vi "GEA3 Write ERD (Rev 2 API).vi"(0 "GEA2 Reference In":refnum<k24>, 1 "# of Tries":u8=5 min=1 step=1, 2 "Read Timeout (ms)":u32=500, 5 "GEA Inputs":T3 {"Destination" format="%.0x"; "Source" format="%.0x"}, 7 "ERD Write Data In":T1 {"ERD Number" format="%.0x"}, 11 "Error In":errorcluster, 13 "Verify ERD Response?":bool=TRUE) -> (4 "GEA2 Reference Out":refnum<k24>, 6 "Raw Data Out":string, 15 "Error Out":errorcluster)   [LabVIEW 2018, in "GEA2_Toolkit.lvlib"]
doc: "This VI writes an array of ERDs with a single command. The data type is used to convert the Data from the type specified to a hexidecimal string before sending it."
uses:
  C:/Users/iallatyp/Desktop/New folder/GEA3/library/GEA2_Toolkit.lvlib
  D:/Common/LabVIEW GEA2 Toolkit/source/GEA3 DLL Source/GeaCommunication.dll
  source/GEA3 DLL Source/GeaCommunication.dll
  type defs/Source_Destination.ctl
  type defs/ERD Write Data In.ctl
  type defs/Data Type.ctl
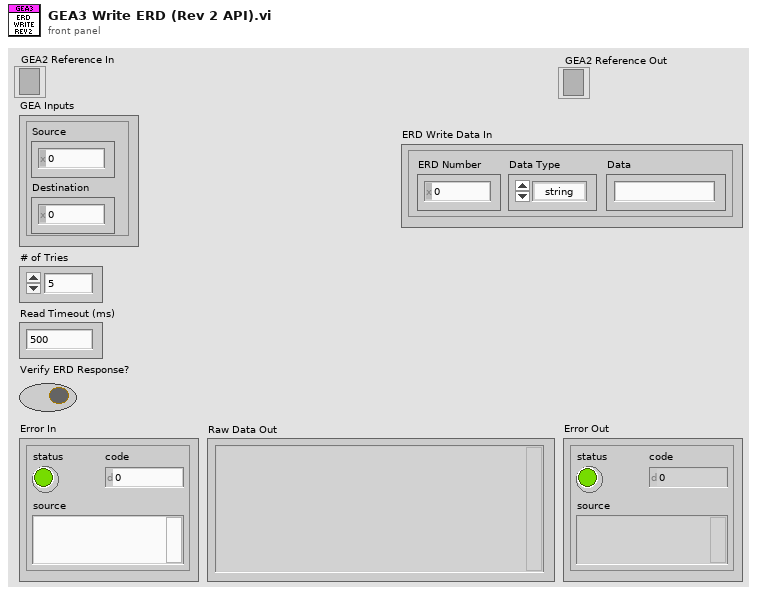
[diagram p1: front panel]
types:
  T1 = typedef "GEA2_Toolkit.lvlib/ERD Write Data In.ctl" = cluster{"ERD Number":u16, "Data Type":T2, "Data":string}
  T2 = typedef "GEA2_Toolkit.lvlib/Data Type.ctl" = enum16{"string", "boolean", "uint8_t", "uint16_t", "uint32_t", "uint64_t", "int8_t", "int16_t", "int32_t", "int64_t"}
  T3 = typedef "GEA2_Toolkit.lvlib/Source_Destination.ctl" = cluster{"Source":u8, "Destination":u8}
  T4 = typedef "GEA2_Toolkit.lvlib/Data In.ctl" = cluster{"Source":u8, "Destination":u8, "Command":u8, "Message":string}
  T5 = typedef "GEA2_Toolkit.lvlib/Data Out.ctl" = cluster{"Source":u8, "Destination":u8, "Command":u8, "Length":u8, "CRC":u16, "Message":string}
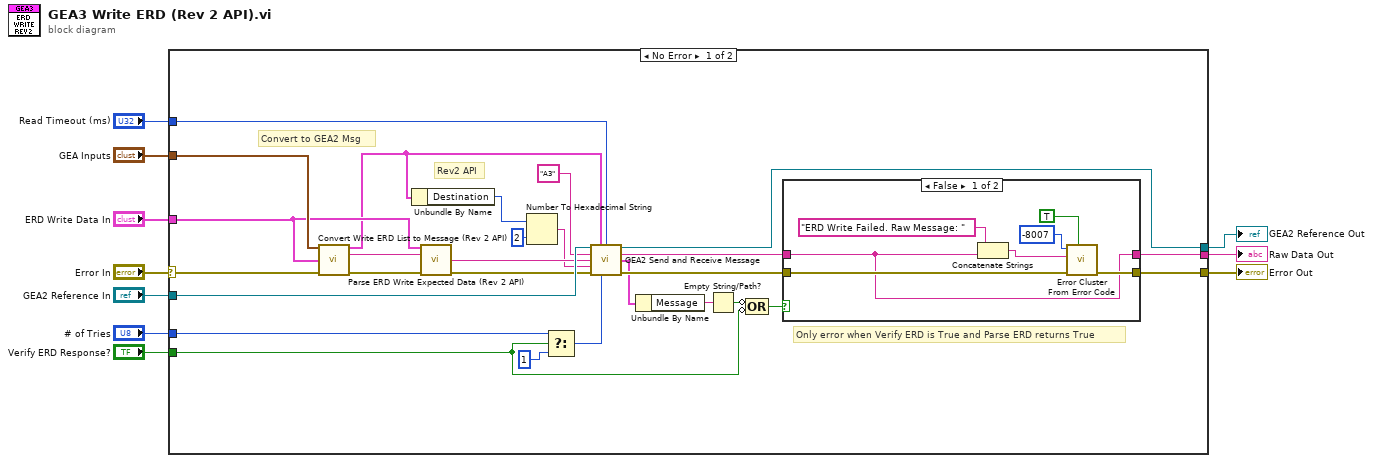
[diagram p0: block diagram]
diagram:
  n1 = case shown="No Error" "Error In" {
    selector: "Error In" -> [w30 w47]
    tunnel: "GEA2 Reference In" -> [w29 w48]
    tunnel: "ERD Write Data In" -> [w28 _]
    tunnel: "Verify ERD Response?" -> [w37 _]
    tunnel: "GEA Inputs" -> [w31 _]
    tunnel: [w33 _] -> w7
    tunnel: [w34 w47] -> w3
    tunnel: "Read Timeout (ms)" -> [w36 _]
    tunnel: "# of Tries" -> [w35 _]
    tunnel: [w32 w48] -> w4
    frame No Error {
      # "Rev2 API"
      # "Only error when Verify ERD is True and Parse ERD returns True"
      # "Convert to GEA2 Msg"
      n2 = call "Convert Write ERD List to Message (Rev 2 API).vi"("GEA Inputs"=w31, "ERD Read Data In"=w28, "Error In"=w30) -> ("GEA Message"=w23:T4, "Request ID"=w11:string, "Error Out"=w26:errorcluster)  [unwired: 10 in]
      n3 = Unbundle By Name(w23) -> ("Destination"=w14:u8)
      n4 = call "Parse ERD Write Expected Data (Rev 2 API).vi"("ERD Write Data In"=w28, "Request ID"=w11, "Error In"=w26) -> ("Expected Data"=w24:string, "Error Out"=w25:errorcluster)  [unwired: 11 in]
      n5 = Number To Hexadecimal String(1:i16 2 ("width (-)"), 2:w14) -> (0:w13:string)
      n6 = Select(t=w35, s=w37, f=u8 1) -> (s? t:f=w19:u8)
      n7 = call "GEA2 Send and Receive Message.vi"("GEA2 Reference In"=w29, "Input Data"=w23, "Read Timeout (ms)"=w36, "Expected Command"="A3", "Expected Data"=w24, "Expected Source"=w13, "Error In"=w25, "# of Tries"=w19) -> ("GEA2 Reference Out"=w32:refnum<k24>, "Raw Data Out"=w21:string, "Converted Data Out"=w18:T5, "Error Out"=w22:errorcluster)  [unwired: 4 in]
      n8 = Unbundle By Name(w18) -> ("Message"=w17:string)
      n9 = Empty String/Path?(string/path=w17) -> (empty?=w16:bool)
      n10 = Compound Arithmetic op=OR(invert w16, invert w37) -> (w27:bool)
      n11 = case shown="False" w27 {
        tunnel: w22 -> [w44 w46]
        tunnel: [w43 w46] -> w34
        tunnel: [w38 w45] -> w33
        tunnel: w21 -> [w38 w45]
        frame False {
          n12 = Concatenate Strings("ERD Write Failed. Raw Message: " ("error message (\"\")"), w38) -> (w39:string)
          n13 = call <vilib>:"Error Cluster From Error Code.vi"("show call chain? (False)"=TRUE, "error in (no error)"=w44, "error message (\"\")"=w39, "error code (0)"=-8007) -> ("error out"=w43:errorcluster)  [unwired: 5 in]
        }
        frame True {
        }
      }
    }
    frame Error {
    }
  }
  "Raw Data Out" <- w7
  "GEA2 Reference Out" <- w4
  "Error Out" <- w3
